vi "FYP_VI_MIDI_Test_KeyScanCode.vi"() -> ()   [LabVIEW 2013]
panel:
  in  "Stop":bool
  out "RShift":bool
  out ";":bool
  out "/":bool
  out "L":bool
  out ".":bool
  out ",":bool
  out "J":bool
  out "M":bool
  out "H":bool
  out "N":bool
  out "G":bool
  out "B":bool
  out "V":bool
  out "D":bool
  out "C":bool
  out "Back/S":bool
  out "X":bool
  out "]/Z":bool
  out "-/CAP":bool
  out "[/Shift":bool
  out "0":bool
  out "P":bool
  out "9":bool
  out "O":bool
  out "I":bool
  out "7":bool
  out "U":bool
  out "6":bool
  out "Y":bool
  out "T":bool
  out "4":bool
  out "R":bool
  out "3":bool
  out "E":bool
  out "2":bool
  out "W":bool
  out "Q":bool
  out "~":bool
  out "Tab":bool
  out "ScanCode":i16
  out "MIDI Note Number":i16
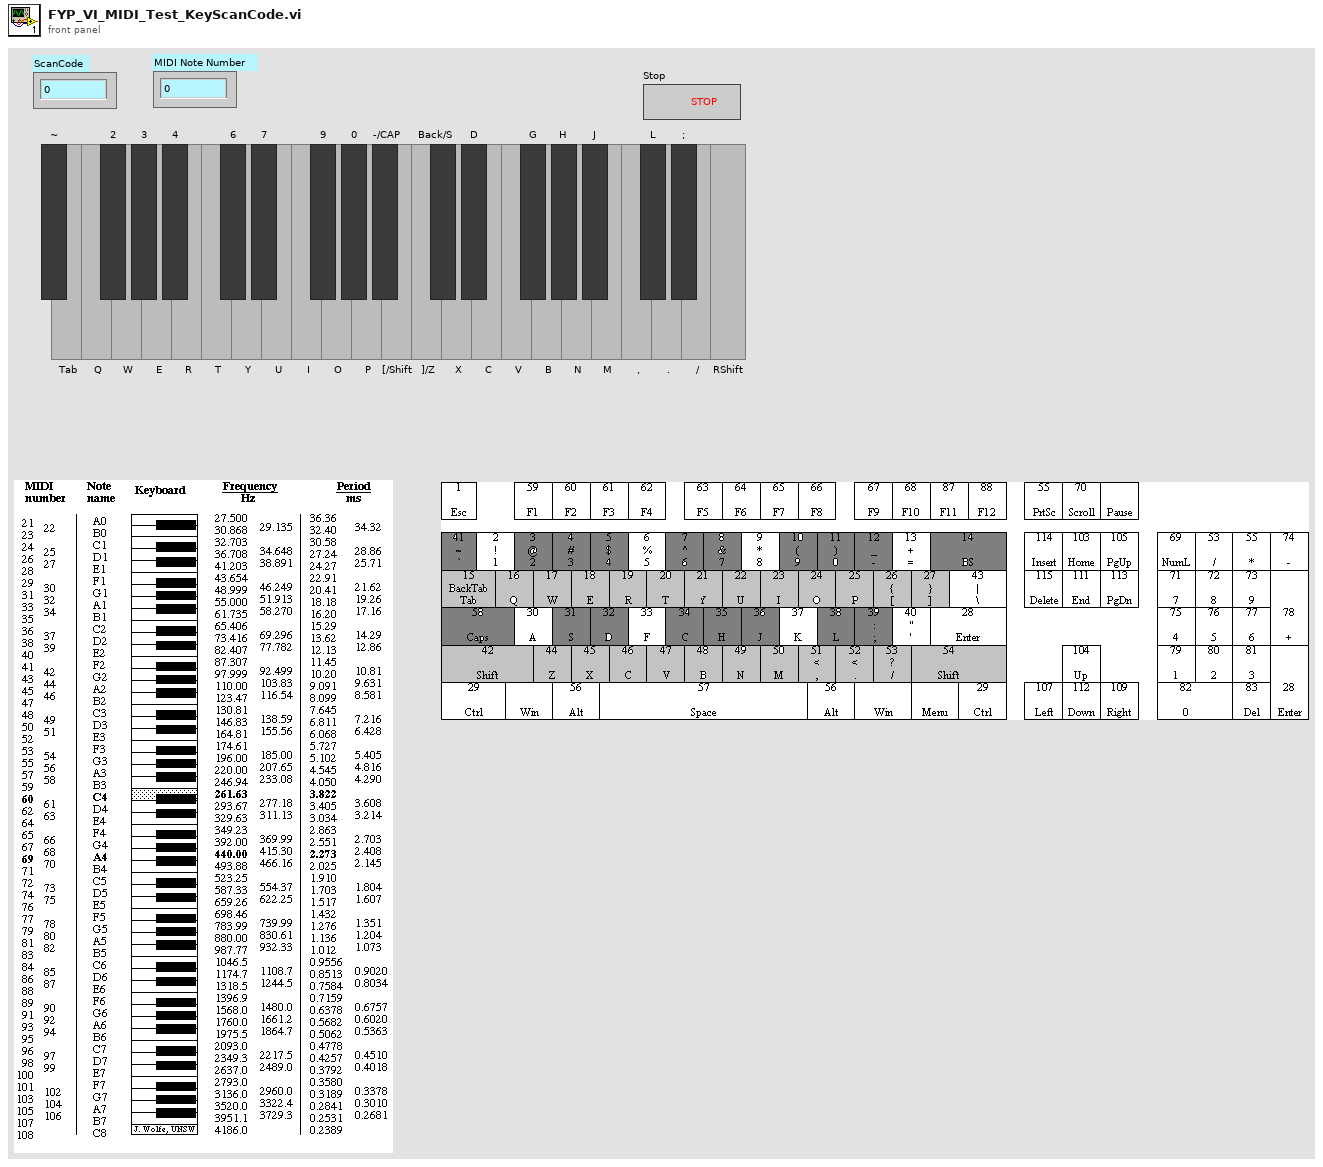
[diagram p1: front panel]
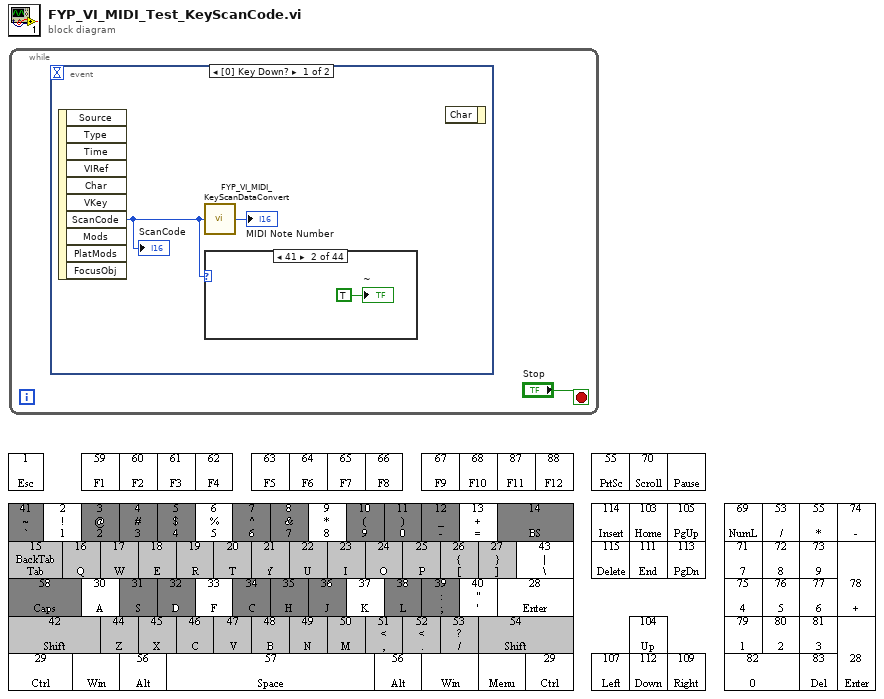
[diagram p0: block diagram]
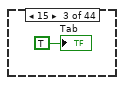
[diagram p3: hidden frame]
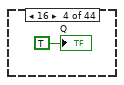
[diagram p4: hidden frame]
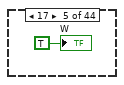
[diagram p5: hidden frame]
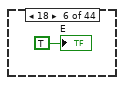
[diagram p6: hidden frame]
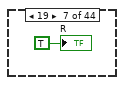
[diagram p7: hidden frame]
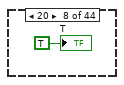
[diagram p8: hidden frame]
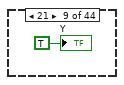
[diagram p9: hidden frame]
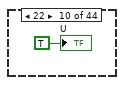
[diagram p10: hidden frame]
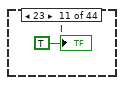
[diagram p11: hidden frame]
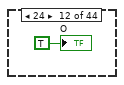
[diagram p12: hidden frame]
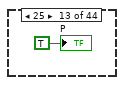
[diagram p13: hidden frame]
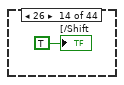
[diagram p14: hidden frame]
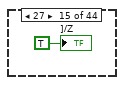
[diagram p15: hidden frame]
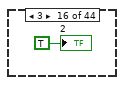
[diagram p16: hidden frame]
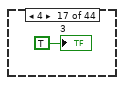
[diagram p17: hidden frame]
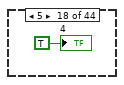
[diagram p18: hidden frame]
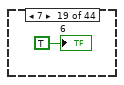
[diagram p19: hidden frame]
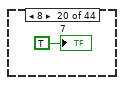
[diagram p20: hidden frame]
diagram:
  n1 = while {
    stop <- "Stop" stop-if-true
    n2 = event shown="[0] Key Down?" {
      selector: _ -> [_ _]
      dyn-events: _ -> [_ _]
      timeout: _ -> [_ _]
      event Key Down? {
        n3 = event-data() -> ("ScanCode"=w2:i16)  [unwired: 1 in, 9 out]
        "ScanCode" <- w2
        n4 = call "FYP_VI_MIDI_KeyScanDataConvert.vi"("KeyScan"=w2) -> ("MIDI Note Number"=→"MIDI Note Number":i16)
        n5 = case shown="41" w2 {
          frame 0, Default {
          }
          frame 41 {
            "~" <- TRUE ("Q")
          }
          frame 15 {
            "Tab" <- TRUE ("Q")
          }
          frame 16 {
            "Q" <- TRUE ("Q")
          }
          frame 17 {
            "W" <- TRUE ("4")
          }
          frame 18 {
            "E" <- TRUE ("4")
          }
          frame 19 {
            "R" <- TRUE ("4")
          }
          frame 20 {
            "T" <- TRUE ("4")
          }
          frame 21 {
            "Y" <- TRUE ("4")
          }
          frame 22 {
            "U" <- TRUE ("4")
          }
          frame 23 {
            "I" <- TRUE ("4")
          }
          frame 24 {
            "O" <- TRUE ("4")
          }
          frame 25 {
            "P" <- TRUE ("4")
          }
          frame 26 {
            "[/Shift" <- TRUE ("4")
          }
          frame 27 {
            "]/Z" <- TRUE ("4")
          }
          frame 3 {
            "2" <- TRUE ("Q")
          }
          frame 4 {
            "3" <- TRUE ("4")
          }
          frame 5 {
            "4" <- TRUE ("4")
          }
          frame 7 {
            "6" <- TRUE ("4")
          }
          frame 8 {
            "7" <- TRUE ("4")
          }
          frame 10 {
            "9" <- TRUE ("4")
          }
          frame 11 {
            "0" <- TRUE ("4")
          }
          frame 12 {
            "-/CAP" <- TRUE ("4")
          }
          frame 14 {
            "Back/S" <- TRUE ("4")
          }
          frame 58 {
            n6 = local write "-/CAP"(TRUE ("4")) -> ()
          }
          frame 42 {
            n7 = local write "[/Shift"(TRUE ("4")) -> ()
          }
          frame 44 {
            n8 = local write "]/Z"(TRUE ("4")) -> ()
          }
          frame 45 {
            "X" <- TRUE ("4")
          }
          frame 46 {
            "C" <- TRUE ("4")
          }
          frame 47 {
            "V" <- TRUE ("4")
          }
          frame 48 {
            "B" <- TRUE ("4")
          }
          frame 49 {
            "N" <- TRUE ("4")
          }
          frame 50 {
            "M" <- TRUE ("4")
          }
          frame 51 {
            "," <- TRUE ("4")
          }
          frame 52 {
            "." <- TRUE ("4")
          }
          frame 53 {
            "/" <- TRUE ("4")
          }
          frame 54 {
            "RShift" <- TRUE ("4")
          }
          frame 31 {
            n9 = local write "Back/S"(TRUE ("4")) -> ()
          }
          frame 32 {
            "D" <- TRUE ("4")
          }
          frame 34 {
            "G" <- TRUE ("4")
          }
          frame 35 {
            "H" <- TRUE ("4")
          }
          frame 36 {
            "J" <- TRUE ("4")
          }
          frame 38 {
            "L" <- TRUE ("4")
          }
          frame 39 {
            ";" <- TRUE ("4")
          }
        }
        n10 = event-data() -> ()  [unwired: 2 in, 1 out]
      }
      event Key Up {
        n11 = event-data() -> ("ScanCode"=w47:i16)  [unwired: 1 in, 7 out]
        n12 = case shown="41" w47 {
          frame 0, Default {
          }
          frame 41 {
            n13 = local write "~"(FALSE ("Q")) -> ()
          }
          frame 15 {
            n14 = local write "Tab"(FALSE ("Q")) -> ()
          }
          frame 16 {
            n15 = local write "Q"(FALSE ("Q")) -> ()
          }
          frame 17 {
            n16 = local write "W"(FALSE ("4")) -> ()
          }
          frame 18 {
            n17 = local write "E"(FALSE ("4")) -> ()
          }
          frame 19 {
            n18 = local write "R"(FALSE ("4")) -> ()
          }
          frame 20 {
            n19 = local write "T"(FALSE ("4")) -> ()
          }
          frame 21 {
            n20 = local write "Y"(FALSE ("4")) -> ()
          }
          frame 22 {
            n21 = local write "U"(FALSE ("4")) -> ()
          }
          frame 23 {
            n22 = local write "I"(FALSE ("4")) -> ()
          }
          frame 24 {
            n23 = local write "O"(FALSE ("4")) -> ()
          }
          frame 25 {
            n24 = local write "P"(FALSE ("4")) -> ()
          }
          frame 26 {
            n25 = local write "[/Shift"(FALSE ("4")) -> ()
          }
          frame 27 {
            n26 = local write "]/Z"(FALSE ("4")) -> ()
          }
          frame 3 {
            n27 = local write "2"(FALSE ("Q")) -> ()
          }
          frame 4 {
            n28 = local write "3"(FALSE ("3")) -> ()
          }
          frame 5 {
            n29 = local write "4"(FALSE ("4")) -> ()
          }
          frame 7 {
            n30 = local write "6"(FALSE ("4")) -> ()
          }
          frame 8 {
            n31 = local write "7"(FALSE ("4")) -> ()
          }
          frame 10 {
            n32 = local write "9"(FALSE ("4")) -> ()
          }
          frame 11 {
            n33 = local write "0"(FALSE ("4")) -> ()
          }
          frame 12 {
            n34 = local write "-/CAP"(FALSE ("4")) -> ()
          }
          frame 14 {
            n35 = local write "Back/S"(FALSE ("4")) -> ()
          }
          frame 58 {
            n36 = local write "-/CAP"(FALSE ("4")) -> ()
          }
          frame 42 {
            n37 = local write "[/Shift"(FALSE ("4")) -> ()
          }
          frame 44 {
            n38 = local write "]/Z"(FALSE ("4")) -> ()
          }
          frame 45 {
            n39 = local write "X"(FALSE ("4")) -> ()
          }
          frame 46 {
            n40 = local write "C"(FALSE ("4")) -> ()
          }
          frame 47 {
            n41 = local write "V"(FALSE ("4")) -> ()
          }
          frame 48 {
            n42 = local write "B"(FALSE ("4")) -> ()
          }
          frame 49 {
            n43 = local write "N"(FALSE ("4")) -> ()
          }
          frame 50 {
            n44 = local write "M"(FALSE ("4")) -> ()
          }
          frame 51 {
            n45 = local write ","(FALSE ("4")) -> ()
          }
          frame 52 {
            n46 = local write "."(FALSE ("4")) -> ()
          }
          frame 53 {
            n47 = local write "/"(FALSE ("4")) -> ()
          }
          frame 54 {
            n48 = local write "RShift"(FALSE ("4")) -> ()
          }
          frame 31 {
            n49 = local write "Back/S"(FALSE ("4")) -> ()
          }
          frame 32 {
            n50 = local write "D"(FALSE ("4")) -> ()
          }
          frame 34 {
            n51 = local write "G"(FALSE ("4")) -> ()
          }
          frame 35 {
            n52 = local write "H"(FALSE ("4")) -> ()
          }
          frame 36 {
            n53 = local write "J"(FALSE ("4")) -> ()
          }
          frame 38 {
            n54 = local write "L"(FALSE ("4")) -> ()
          }
          frame 39 {
            n55 = local write ";"(FALSE ("4")) -> ()
          }
        }
      }
    }
  }
